vi "AuMT8852B Check Integer Range.vi"(5 "Value (0)":i32, 6 "Check IVI flag first? (T)":bool=TRUE, 7 "Set/Get (Set)":enum16{"Set", "Get"}(ring), 8 "error in (no error)":errorcluster, 9 "Lower limit (-1)":i32=-1, 10 "Upper limit (1)":i32=1, 11 "VISA session":refnum<visa-resource-name>) -> (0 "error out":errorcluster, 3 "VISA session out":refnum<visa-resource-name>)   [LabVIEW 2017]
doc: "Anritsu MT8852B Bluetooth Tester\n\nReturns an error if the value is outside the specified range.\n\nINPUTS\nSet/Get - range checking will be skipped if this control is Get.\nValue - value to be checked.\nUpper limit, lower limit - valid range for the value (the limits are also valid values).\nCheck IVI flag first? - if True, range checking will not be done if the IVI range-checking flag is off. If False, this VI will not check the IVI flag."
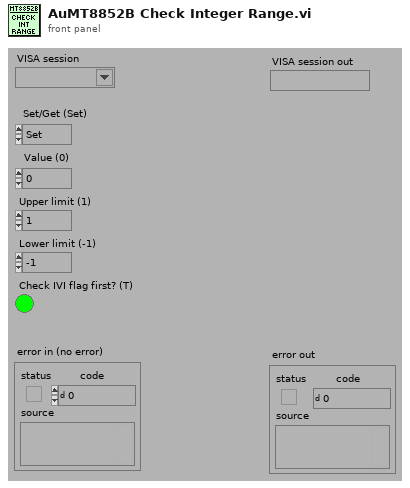
[diagram p1: front panel]
types:
  T1 = enum16{"Simulate", "Range check", "Cache", "Query instrument status"}
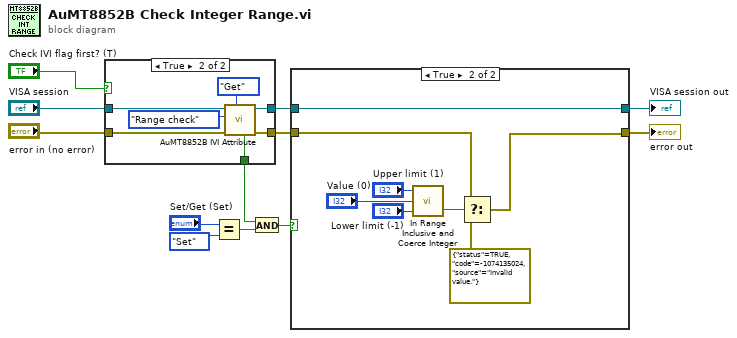
[diagram p0: block diagram]
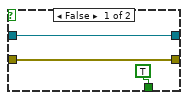
[diagram p2: hidden frame]
diagram:
  n1 = case shown="True" "Check IVI flag first? (T)" {
    tunnel: [w13 w22] -> w10
    tunnel: [w14 w21] -> w9
    tunnel: "VISA session" -> [w13 w20]
    tunnel: "error in (no error)" -> [w14 w19]
    tunnel: [TRUE ("Value out") w16] -> w2
    frame False {
    }
    frame True {
      n2 = call <instrlib>:"AuMT8852B IVI Attribute.vi"("Set/Get (Set)"=enum16{"Set", "Get"}."Get", "error in (no error)"=w19, "Flag (Simulate)"=T1."Range check", "VISA session"=w20) -> ("error out"=w21:errorcluster, "VISA session out"=w22:refnum<visa-resource-name>, "Value out"=w16:bool)  [unwired: 5 in]
    }
  }
  n3 = Equal?(x="Set/Get (Set)", y=enum16{"Set", "Get"}."Set") -> (x = y?=w3:bool)
  n4 = And(x=w2, y=w3) -> (x .and. y?=w4:bool)
  n5 = case shown="True" w4 {
    tunnel: [w24 w29] -> w12
    tunnel: w10 -> [w24 w29]
    tunnel: [w23 w25] -> w11
    tunnel: w9 -> [w23 w26]
    frame False {
    }
    frame True {
      n6 = call <instrlib>:"In Range Inclusive and Coerce Integer.vi"("Lower limit (-1)"="Lower limit (-1)", "X (0)"="Value (0)", "Upper limit (1)"="Upper limit (1)") -> ("In range?"=w28:bool)  [unwired: 1 out]
      n7 = Select(t=w26, s=w28, f=errorcluster {"status"=TRUE, "code"=-1074135024, "source"="Invalid value."}) -> (s? t:f=w25:errorcluster)
    }
  }
  "VISA session out" <- w12
  "error out" <- w11
